vi "Calibration page.vi"(0 "sensor data array":dbl[](array[numeric]), 1 "sensor thr array":dbl[](array[numeric]), 2 "counting role":T1(ring), 3 "sensor1 array":dbl[](array[numeric]), 4 "curv array in":dbl[](array[numeric]), 5 "count in":dbl, 6 "sensor2 array":dbl[](array[numeric]), 7 "sensor3 array":dbl[](array[numeric]), 8 "curv sw info":dbl[](array[numeric]), 9 "capture":bool, 10 "cyrv avg array in":dbl[][][](array[numeric]), 11 "error in":errorcluster, 16 "sen plt num":i32) -> (12 "Left Sidewall":bool, 13 "cyrv avg array out":dbl[][][](array[numeric]), 14 "Right Sidewall":bool, 15 "curv sit":bool, 17 "Boolean Rectangle 5":bool, 18 "Col Curve":dbl[](array[numeric]), 19 "error out":errorcluster, 20 "Curvness Sensors Graph":dynamicdata(graph), 21 "SideWall Sensors Graph":dynamicdata(graph), 22 "sensor1 array out":dbl[](array[numeric]), 23 "curv array out":dbl[](array[numeric]), 24 "sensor2 array out":dbl[](array[numeric]), 25 "sensor3 array out":dbl[](array[numeric]), 26 "capture":bool, 27 "Pallet CURV (mm)":dbl format="%#_2g")   [LabVIEW 2019]
uses:
  <vilib>/measure/mamon.llb/Trigger Detection for 1 Channel.vi
  <vilib>/measure/NI_MAPro.lvlib
panel:
  out "curv array in 2":dbl[](array[numeric])
  out "subarray 3":dbl[](array[numeric])
  out "subarray 2":dbl[](array[numeric])
  out "Boolean":bool
  out "subarray":dbl[](array[numeric])
  out "x+y 3":dbl
  out "x+y 2":dbl
  out "x+y":dbl
  in  "bias":dbl format="%#_13g"
  out "sesor3-2 dis":dbl
  out "sensor2-2 dis":dbl
  out "sensor1-2 dis":dbl
  out "Numeric 3":i32=1
  out "Numeric 2":i32=1
  out "sensor3 dis":dbl
  out "sensor2 dis":dbl
  out "sensor1 dis":dbl
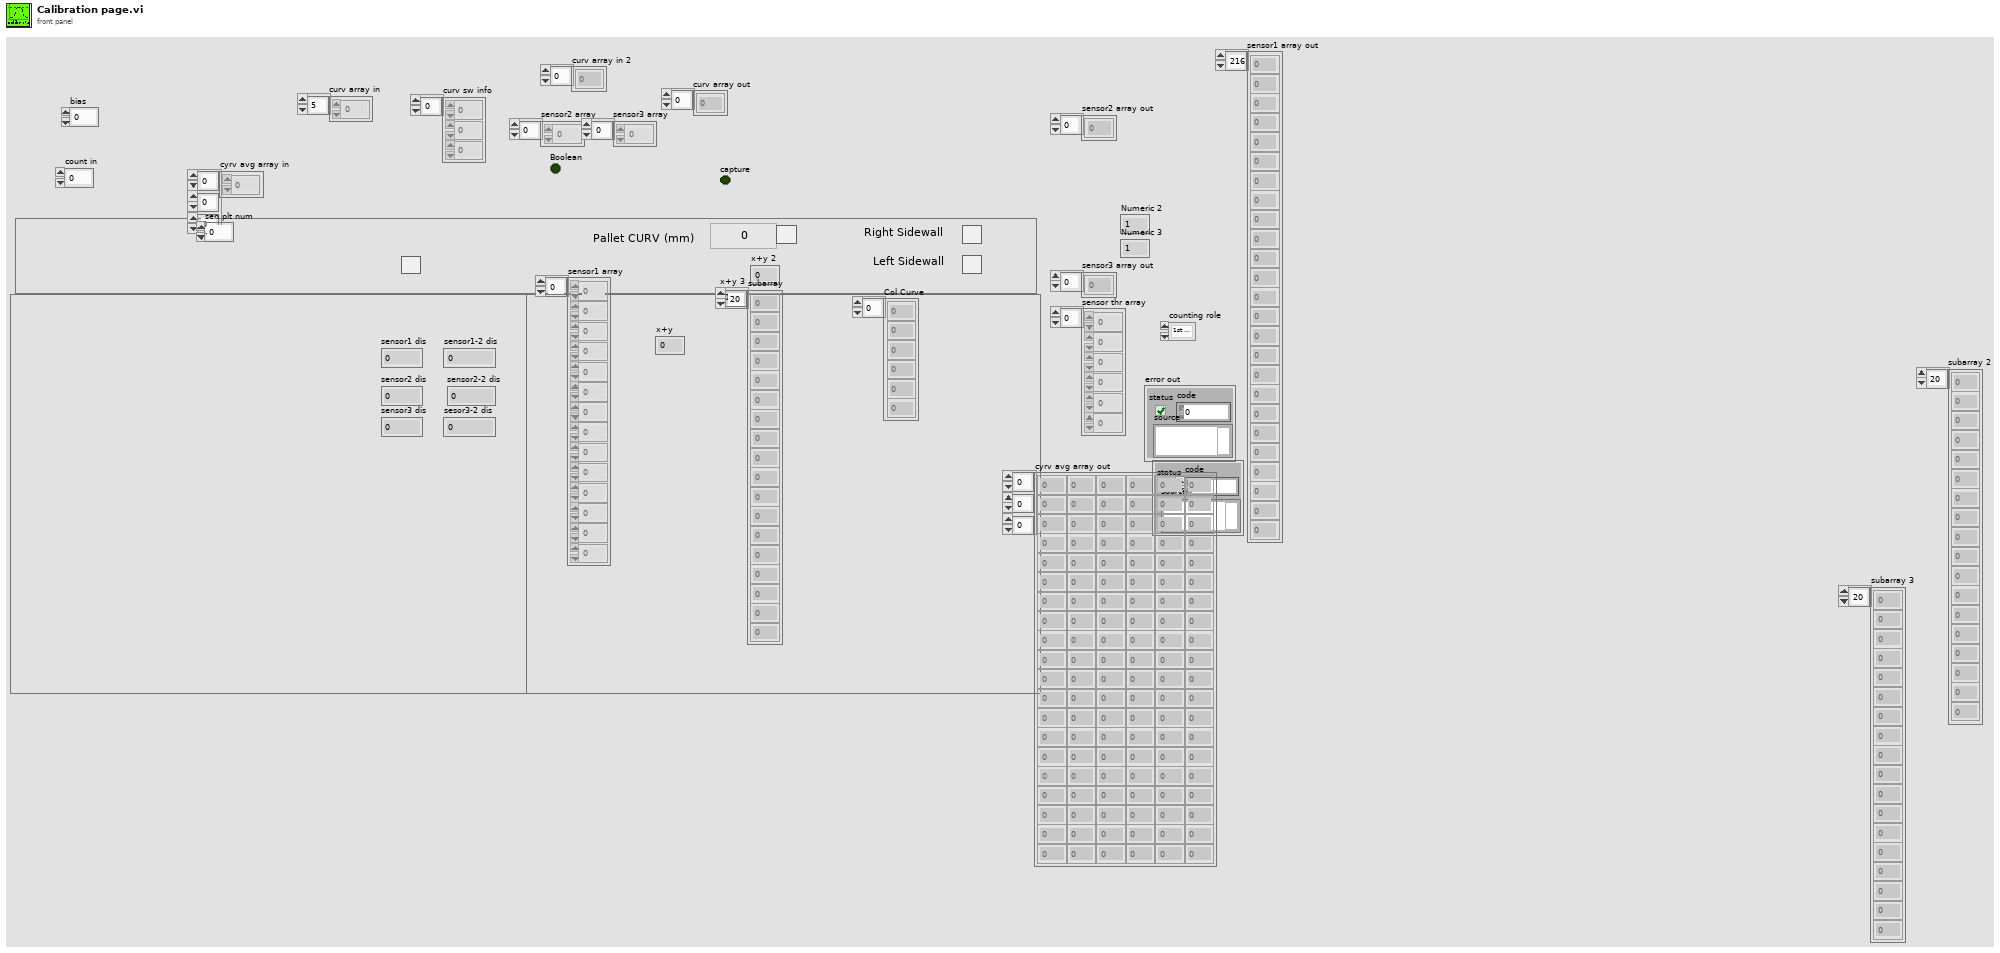
[diagram p1: front panel]
types:
  T1 = enum16{"1st sensor", "2nd sensor", "3rd sensor", "1st+2nd", "1st+3rd", "2nd+3rd", "1st+2nd+3rd"}
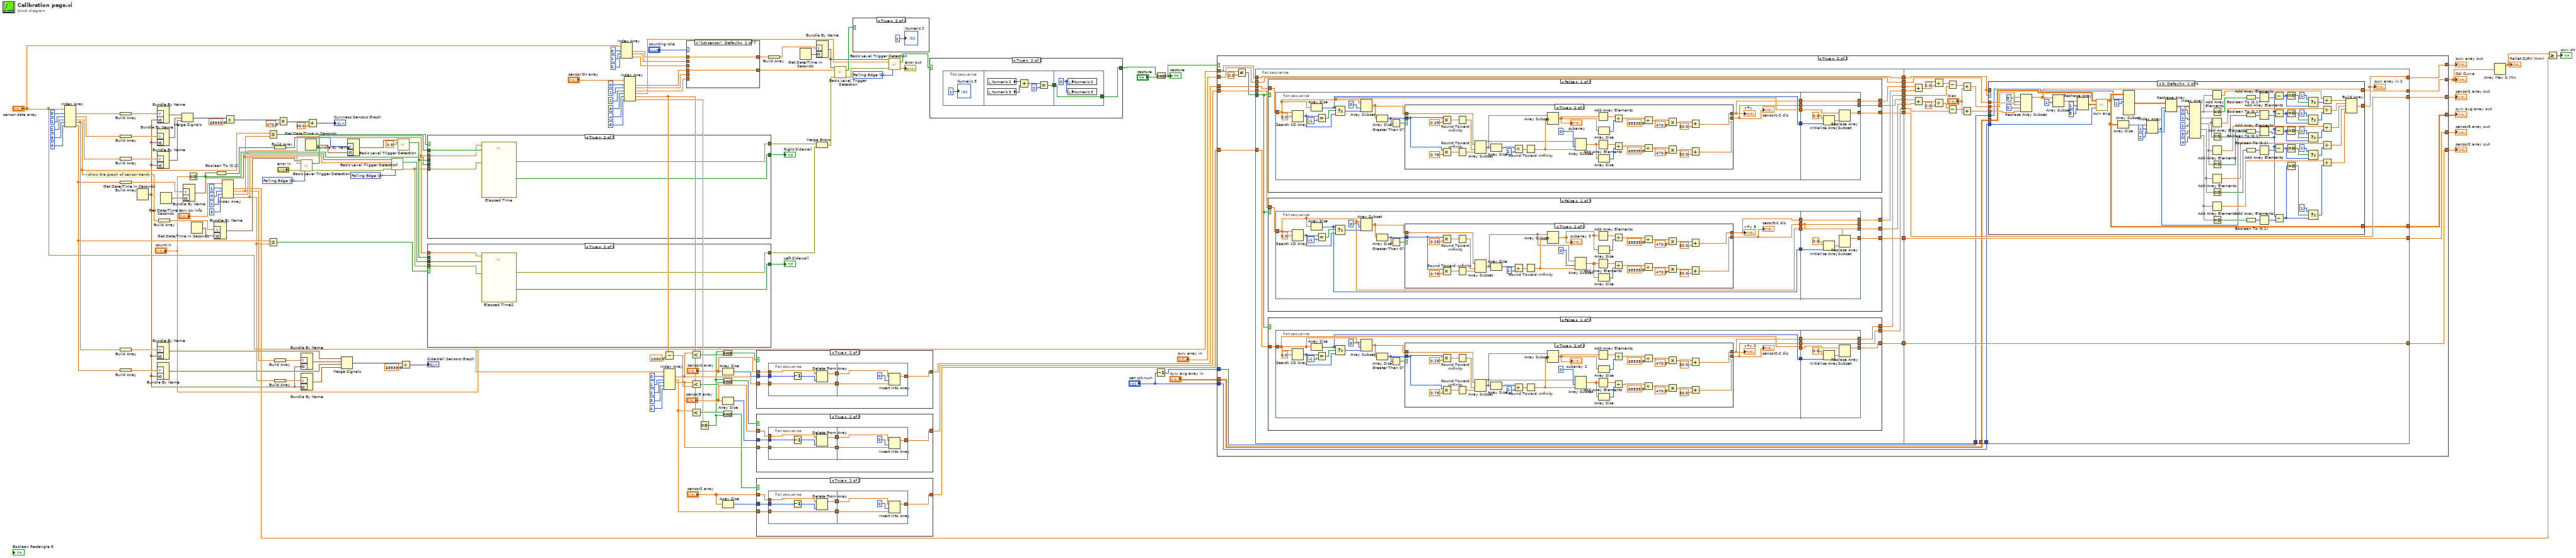
[diagram p0: block diagram]
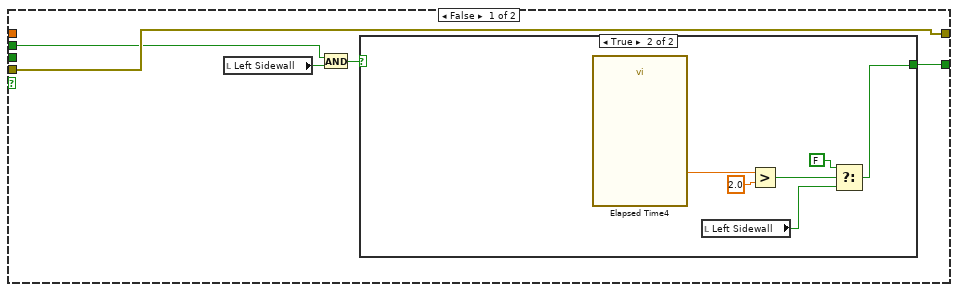
[diagram p5: hidden frame]
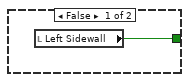
[diagram p6: hidden frame]
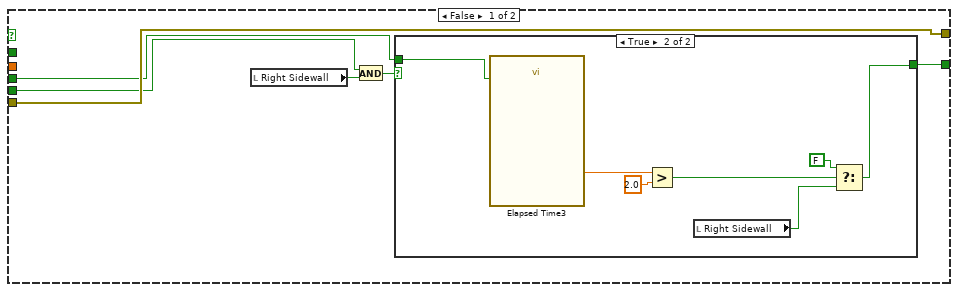
[diagram p7: hidden frame]
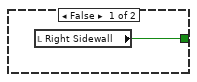
[diagram p8: hidden frame]
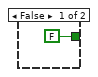
[diagram p9: hidden frame]
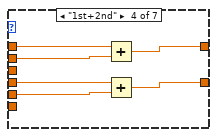
[diagram p13: hidden frame]
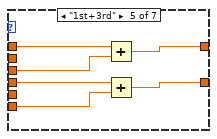
[diagram p14: hidden frame]
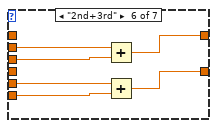
[diagram p15: hidden frame]
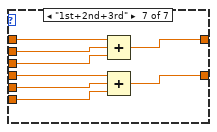
[diagram p16: hidden frame]
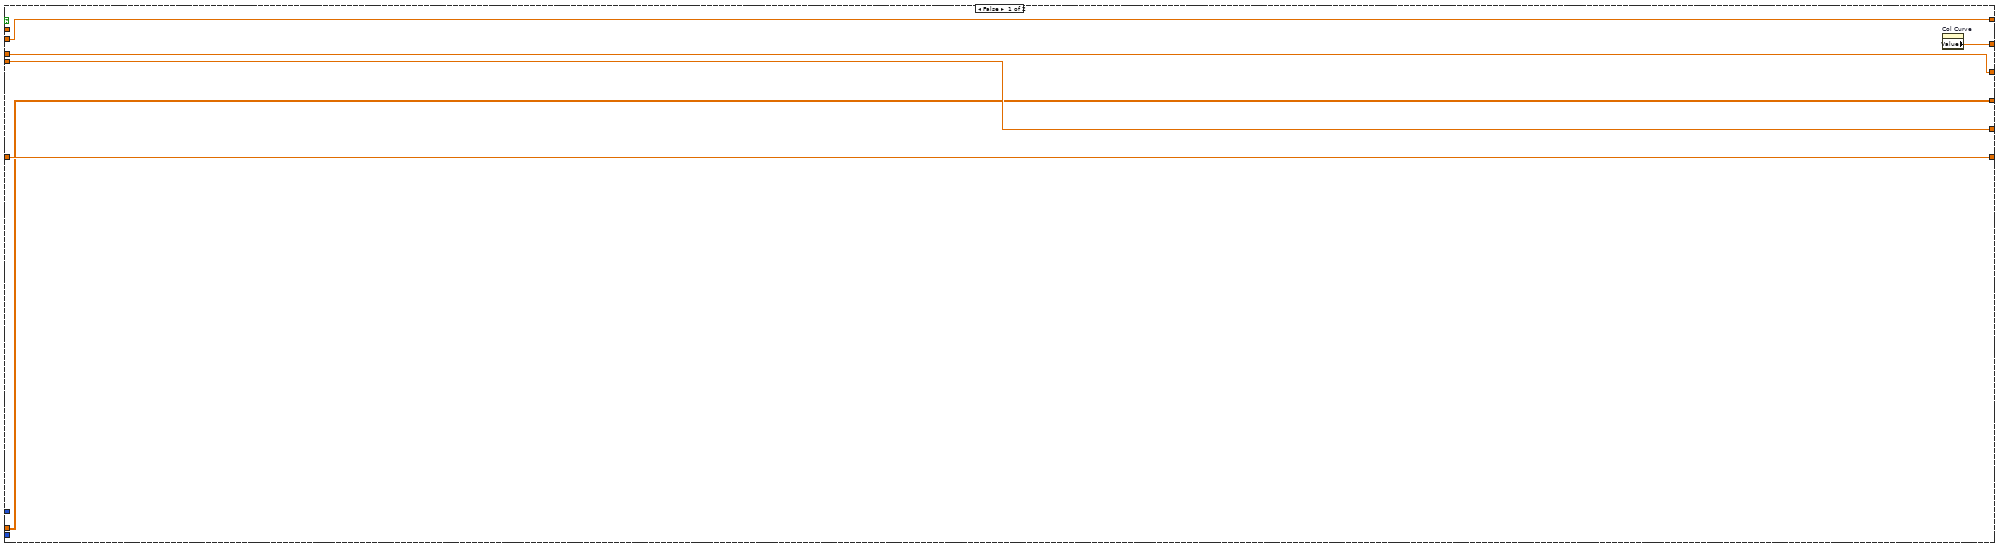
[diagram p17: hidden frame]
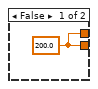
[diagram p18: hidden frame]
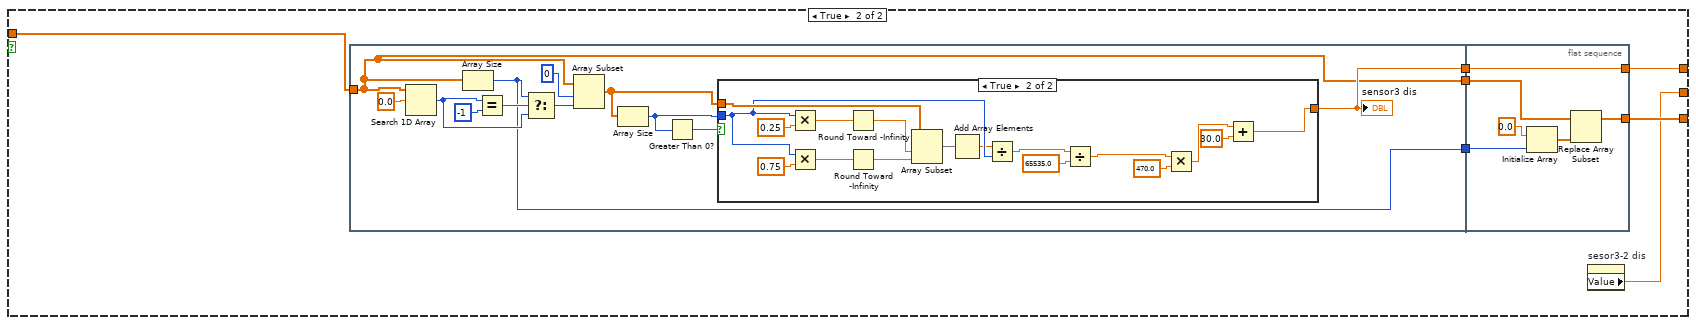
[diagram p19: hidden frame]
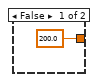
[diagram p20: hidden frame]
diagram:
  w38 = u16 0 items=["Falling Edge", "Rising Edge"] ("trigger slope")
  w39 = u16 0 items=["Falling Edge", "Rising Edge"] ("trigger slope")
  w100 = u16 0 items=["Falling Edge", "Rising Edge"] ("trigger slope")
  # "show the graph of sensor trend"
  n1 = Index Array(array="sensor data array", index #1=0 ("index"), index #2=1 ("index"), index #3=2 ("index"), index #4=3 ("index"), index #5=4 ("index")) -> (element #1=w136:dbl, element #2=w134:dbl, element #3=w132:dbl, element #4=w69:dbl, element #5=w68:dbl)
  n2 = Build Array(w136) -> (w135:dbl[])
  n3 = Build Array(w134) -> (w133:dbl[])
  n4 = Build Array(w132) -> (w131:dbl[])
  n5 = Build Array(w68) -> (w67:dbl[])
  n6 = Build Array(w69) -> (w130:dbl[])
  n7 = Build Array(w68) -> (w129:dbl[])
  n8 = Get Date/Time In Seconds() -> (seconds since 1Jan1904=w12:timestamp)
  n9 = Bundle By Name("Y"=w135, "t0"=w12) -> (w123:waveform(dbl))  [unwired: 1 in]
  n10 = Bundle By Name("Y"=w133, "t0"=w12) -> (w144:waveform(dbl))  [unwired: 1 in]
  n11 = Bundle By Name("Y"=w131, "t0"=w12) -> (w143:waveform(dbl))  [unwired: 1 in]
  n12 = Bundle By Name("Y"=w130, "t0"=w12) -> (w142:waveform(dbl))  [unwired: 1 in]
  n13 = Bundle By Name("Y"=w129, "t0"=w12) -> (w17:waveform(dbl))  [unwired: 1 in]
  n14 = Build Array(w69) -> (w70:dbl[])
  n15 = Get Date/Time In Seconds() -> (seconds since 1Jan1904=w92:timestamp)
  n16 = Merge Signals(w123, w144, w143) -> (w11:dynamicdata)
  n17 = Bundle By Name("Y"=w67, "t0"=w92) -> (w93:waveform(dbl))  [unwired: 1 in]
  n18 = Equal To 0?(x="count in") -> (x = 0?=w28:bool)
  n19 = Get Date/Time In Seconds() -> (seconds since 1Jan1904=w96:timestamp)
  n20 = Bundle By Name("Y"=w70, "t0"=w96) -> (w95:waveform(dbl))  [unwired: 1 in]
  n21 = Boolean To (0,1)(Boolean=w28) -> (0, 1=w32:i16)
  n22 = Index Array(array="curv sw info", index #1=1 ("index"), index #2=0 ("index"), index #3=2 ("index"), index #4=3 ("index")) -> (element #1=w43:dbl, element #2=w19:dbl, element #3=w66:dbl, element #4=w14:dbl)
  n23 = Divide(x=w11, y=65535.0) -> (x/y=w26:dynamicdata)
  n24 = Less Or Equal?(x=w69, y=w19) -> (x <= y?=w98:bool)
  n25 = Less Or Equal?(x=w68, y=w14) -> (x <= y?=w97:bool)
  n26 = Build Array(w32) -> (w31:i16[])
  n27 = Build Array(w19) -> (w18:dbl[])
  n28 = Build Array(w14) -> (w15:dbl[])
  n29 = Multiply(x=w26, y=470.0) -> (x*y=w27:dynamicdata)
  n30 = call-poly <vilib>:"Basic Level Trigger Detection.vi"("signal in"=w95, "level"=w19, "error in (no error)"="error in", "trigger slope"=w39) -> ("trigger detected?"=w94:bool, "error out"=w89:errorcluster)  [unwired: 9 in, 1 out]
  n31 = Bundle By Name("Y"=w18, "t0"=w12) -> (w16:waveform(dbl))  [unwired: 1 in]
  n32 = Bundle By Name("Y"=w15, "t0"=w12) -> (w13:waveform(dbl))  [unwired: 1 in]
  n33 = Get Date/Time In Seconds() -> (seconds since 1Jan1904=w33:timestamp)
  n34 = Add(x=w27, y=30.0) -> (x+y=→"Curvness Sensors Graph":dynamicdata)
  n35 = Merge Signals(w142, w16, w17, w13) -> (w21:dynamicdata)
  n36 = Bundle By Name("Y"=w31, "t0"=w33) -> (w34:waveform(i16))  [unwired: 1 in]
  n37 = call-poly <vilib>:"Basic Level Trigger Detection.vi"("signal in"=w93, "level"=w14, "error in (no error)"=w89, "trigger slope"=w38) -> ("trigger detected?"=w91:bool, "error out"=w51:errorcluster)  [unwired: 9 in, 1 out]
  n38 = call-poly <vilib>:"Basic Level Trigger Detection.vi"("signal in"=w34, "level"=0.5) -> ("trigger detected?"=w29:bool)  [unwired: 11 in, 2 out]
  n39 = Divide(x=w21, y=65535.0) -> (x/y=→"SideWall Sensors Graph":dynamicdata)
  n40 = case shown="True" w98 {
    tunnel: w94 -> [_ w163]
    tunnel: w66 -> [_ w162]
    tunnel: w51 -> [w150 w161]
    tunnel: [w150 w160] -> w50
    tunnel: [w149 w159] -> w37
    tunnel: w29 -> [w148 _]
    tunnel: w28 -> [w146 _]
    frame False {
      n41 = local read "Right Sidewall"() -> (w147:bool)
      n42 = And(x=w146, y=w147) -> (x .and. y?=w145:bool)
      n43 = case shown="True" w145 {
        tunnel: [w151 w153] -> w149
        tunnel: w148 -> [_ w152]
        frame False {
          n44 = local read "Right Sidewall"() -> (w151:bool)
        }
        frame True {
          n45 = call "Elapsed Time3"("Reset"=w152) -> ("Elapsed Time (s)"=w158:dbl)  [unwired: 11 in, 7 out]
          n46 = Greater?(x=w158, y=2.0) -> (0:w156:bool)
          n47 = local read "Right Sidewall"() -> (w154:bool)
          n48 = Select(t=FALSE, s=w156, f=w154) -> (s? t:f=w153:bool)
        }
      }
    }
    frame True {
      n49 = call "Elapsed Time"("Time Target (s)"=w162, "Reset"=w163, "error in (no error)"=w161) -> ("Time has Elapsed"=w159:bool, "error out"=w160:errorcluster)  [unwired: 9 in, 6 out]
    }
  }
  "Right Sidewall" <- w37
  n50 = case shown="True" w97 {
    tunnel: w91 -> [_ w180]
    tunnel: w66 -> [_ w179]
    tunnel: w51 -> [w168 w178]
    tunnel: [w168 w177] -> w49
    tunnel: [w167 w176] -> w36
    tunnel: w29 -> [w165 _]
    frame False {
      n51 = local read "Left Sidewall"() -> (w166:bool)
      n52 = And(x=w165, y=w166) -> (x .and. y?=w164:bool)
      n53 = case shown="True" w164 {
        tunnel: [w169 w170] -> w167
        frame False {
          n54 = local read "Left Sidewall"() -> (w169:bool)
        }
        frame True {
          n55 = call "Elapsed Time4"() -> ("Elapsed Time (s)"=w171:dbl)  [unwired: 12 in, 7 out]
          n56 = local read "Left Sidewall"() -> (w172:bool)
          n57 = Greater?(x=w171, y=2.0) -> (0:w174:bool)
          n58 = Select(t=FALSE, s=w174, f=w172) -> (s? t:f=w170:bool)
        }
      }
    }
    frame True {
      n59 = call "Elapsed Time2"("Time Target (s)"=w179, "Reset"=w180, "error in (no error)"=w178) -> ("Time has Elapsed"=w176:bool, "error out"=w177:errorcluster)  [unwired: 9 in, 6 out]
    }
  }
  "Left Sidewall" <- w36
  n60 = Index Array(array="sensor data array", index #1=0 ("index"), index #2=1 ("index"), index #3=2 ("index")) -> (element #1=w111:dbl, element #2=w110:dbl, element #3=w109:dbl)
  n61 = Index Array(array="sensor thr array", index #1=0 ("index"), index #2=1 ("index"), index #3=2 ("index"), index #4=3 ("index"), index #5=4 ("index"), index #6=6 ("index")) -> (element #1=w117:dbl, element #2=w116:dbl, element #3=w115:dbl, element #4=w56:dbl, element #5=w55:dbl, element #6=w9:dbl)
  n62 = Subtract(x=w55, y=1000.0) -> (x-y=w53:dbl)
  n63 = Index Array(array="sensor data array", index #1=0 ("index"), index #2=1 ("index"), index #3=2 ("index"), index #4=3 ("index"), index #5=4 ("index")) -> (element #1=w77:dbl, element #2=w76:dbl, element #3=w75:dbl)  [unwired: 2 out]
  n64 = case shown="\"1st sensor\", Default" "counting role" {
    tunnel: w111 -> [w182 _ _ w190 w198 _ w212]
    tunnel: w117 -> [w181 _ _ w191 w196 _ w209]
    tunnel: w110 -> [_ w184 _ w192 _ w204 w211]
    tunnel: w109 -> [_ _ w186 _ w197 w203 w210]
    tunnel: w116 -> [_ w183 _ w189 _ w202 w208]
    tunnel: w115 -> [_ _ w185 _ w195 w201 w207]
    tunnel: [w182 w184 w186 w188 w194 w200 w206] -> w105
    tunnel: [w181 w183 w185 w187 w193 w199 w205] -> w106
    frame "1st sensor", Default {
    }
    frame "2nd sensor" {
    }
    frame "3rd sensor" {
    }
    frame "1st+2nd" {
      n65 = Add(x=w190, y=w192) -> (x+y=w188:dbl)
      n66 = Add(x=w191, y=w189) -> (x+y=w187:dbl)
    }
    frame "1st+3rd" {
      n67 = Add(x=w198, y=w197) -> (x+y=w194:dbl)
      n68 = Add(x=w196, y=w195) -> (x+y=w193:dbl)
    }
    frame "2nd+3rd" {
      n69 = Add(x=w204, y=w203) -> (x+y=w200:dbl)
      n70 = Add(x=w202, y=w201) -> (x+y=w199:dbl)
    }
    frame "1st+2nd+3rd" {
      n71 = Compound Arithmetic op=ADD(w212, w211, w210) -> (w206:dbl)
      n72 = Compound Arithmetic op=ADD(w209, w208, w207) -> (w205:dbl)
    }
  }
  n73 = Less?(x=w77, y=w55) -> (x < y?=w8:bool)
  n74 = Less?(x=w75, y=w53) -> (x < y?=w4:bool)
  n75 = Less?(x=w76, y=w55) -> (x < y?=w6:bool)
  n76 = Equal To 0?(x=w9) -> (x = 0?=w3:bool)
  n77 = And(x=w3, y=w8) -> (x .and. y?=w7:bool)
  n78 = And(x=w3, y=w4) -> (x .and. y?=w2:bool)
  n79 = And(x=w6, y=w3) -> (x .and. y?=w5:bool)
  n80 = Array Size(array="sensor1 array") -> (size(s)=w81:i32)
  n81 = Array Size(array="sensor3 array") -> (size(s)=w78:i32)
  n82 = Array Size(array="sensor2 array") -> (size(s)=w80:i32)
  n83 = case shown="True" w7 {
    tunnel: w77 -> [_ w214]
    tunnel: "sensor1 array" -> [w213 w219]
    tunnel: w81 -> [_ w218]
    tunnel: [w213 w216] -> w62
    frame False {
    }
    frame True {
      n84 = flat-sequence {
        tunnel: w219 -> [w224]
        tunnel: w218 -> [w223]
        tunnel: [w221] -> w217
        tunnel: [w220] -> w215
        tunnel: w214 -> [w220]
        tunnel: [w228] -> w216
        tunnel: w215 -> [w225]
        tunnel: w217 -> [w227]
        frame #0 {
          n85 = Decrement(x=w223) -> (x-1=w222:i32)
          n86 = Delete From Array(array=w224, index=w222) -> (array with subset deleted=w221:dbl[])  [unwired: 1 in, 1 out]
        }
        frame #1 {
          n87 = Insert Into Array(array=w227, index=0, new element=w225) -> (w228:dbl[])
        }
      }
    }
  }
  n88 = case shown="True" w2 {
    tunnel: w75 -> [_ w235]
    tunnel: "sensor3 array" -> [w229 w234]
    tunnel: w78 -> [_ w233]
    tunnel: [w229 w230] -> w60
    frame False {
    }
    frame True {
      n89 = flat-sequence {
        tunnel: w235 -> [w236]
        tunnel: w234 -> [w239]
        tunnel: w233 -> [w238]
        tunnel: [w237] -> w232
        tunnel: [w236] -> w231
        tunnel: w232 -> [w243]
        tunnel: w231 -> [w242]
        tunnel: [w241] -> w230
        frame #0 {
          n90 = Decrement(x=w238) -> (x-1=w240:i32)
          n91 = Delete From Array(array=w239, index=w240) -> (array with subset deleted=w237:dbl[])  [unwired: 1 in, 1 out]
        }
        frame #1 {
          n92 = Insert Into Array(array=w243, index=0, new element=w242) -> (w241:dbl[])
        }
      }
    }
  }
  n93 = case shown="True" w5 {
    tunnel: w76 -> [_ w251]
    tunnel: "sensor2 array" -> [w245 w250]
    tunnel: w80 -> [_ w249]
    tunnel: [w245 w246] -> w61
    frame False {
    }
    frame True {
      n94 = flat-sequence {
        tunnel: w251 -> [w252]
        tunnel: w250 -> [w255]
        tunnel: w249 -> [w254]
        tunnel: [w253] -> w248
        tunnel: [w252] -> w247
        tunnel: w248 -> [w259]
        tunnel: w247 -> [w258]
        tunnel: [w257] -> w246
        frame #0 {
          n95 = Decrement(x=w254) -> (x-1=w256:i32)
          n96 = Delete From Array(array=w255, index=w256) -> (array with subset deleted=w253:dbl[])  [unwired: 1 in, 1 out]
        }
        frame #1 {
          n97 = Insert Into Array(array=w259, index=0, new element=w258) -> (w257:dbl[])
        }
      }
    }
  }
  n98 = Build Array(w105) -> (w108:dbl[])
  n99 = Get Date/Time In Seconds() -> (seconds since 1Jan1904=w107:timestamp)
  n100 = Bundle By Name("Y"=w108, "t0"=w107) -> (w104:waveform(dbl))  [unwired: 1 in]
  n101 = Merge Errors(w50, w49) -> (w48:errorcluster)
  n102 = call-poly <vilib>:"Basic Level Trigger Detection.vi"("signal in"=w104, "level"=w106, "error in (no error)"=w48) -> ("trigger detected?"=w103:bool, "error out"=w101:errorcluster)  [unwired: 10 in, 1 out]
  n103 = case shown="True" w103 {
    frame False {
    }
    frame True {
      "Numeric 2" <- 1
    }
  }
  n104 = call-poly <vilib>:"Basic Level Trigger Detection.vi"("signal in"=w104, "level"=w56, "error in (no error)"=w101, "trigger slope"=w100) -> ("trigger detected?"=w102:bool, "error out"=→"error out":errorcluster)  [unwired: 9 in, 1 out]
  n105 = case shown="True" w102 {
    tunnel: [FALSE w264] -> w88
    frame False {
    }
    frame True {
      n106 = flat-sequence {
        tunnel: [w266] -> w263
        tunnel: [w272] -> w264
        tunnel: w263 -> [w272]
        frame #0 {
          "Numeric 3" <- 1
        }
        frame #1 {
          n107 = local read "Numeric 2"() -> (w270:i32)
          n108 = local read "Numeric 3"() -> (w269:i32)
          n109 = Add(x=w270, y=w269) -> (x+y=w268:i32)
          n110 = Equal?(x=w268, y=2) -> (x = y?=w266:bool)
        }
        frame #2 {
          w271 = 0 ("Numeric")
          n111 = local write "Numeric 2"(w271) -> ()
          n112 = local write "Numeric 3"(w271) -> ()
        }
      }
    }
  }
  n113 = Decrement(x="sen plt num") -> (x-1=w42:i32)
  n114 = And(x=w88, y="capture") -> (x .and. y?=w84:bool)
  "capture" <- w84
  n115 = case shown="True" w84 {
    tunnel: "count in" -> [_ w302]
    tunnel: "curv array in" -> [w278 w305]
    tunnel: [w278 w298] -> w83
    tunnel: w62 -> [w277 w301]
    tunnel: w61 -> [w276 w297]
    tunnel: w60 -> [w275 w296]
    tunnel: [w277 w288] -> w65
    tunnel: [w276 w286] -> w64
    tunnel: [w275 w284] -> w63
    tunnel: "cyrv avg array in" -> [w274 w283]
    tunnel: [w274 w282] -> w45
    tunnel: "sen plt num" -> [_ w281]
    tunnel: w42 -> [_ w279]
    tunnel: [w273 w280] -> w41
    frame False {
      n116 = property on="Col Curve" class="Arr (strict)"() -> ("Value"=w273:dbl[])  [unwired: 2 in, 2 out]
    }
    frame True {
      n117 = Not Equal?(x=w302, y=0.0) -> (x != y?=w303:bool)
      n118 = flat-sequence {
        tunnel: w302 -> [w320]
        tunnel: w305 -> [w319]
        tunnel: w303 -> [w316]
        tunnel: w301 -> [w318]
        tunnel: [w320] -> w300
        tunnel: [w319] -> w299
        tunnel: w297 -> [w317]
        tunnel: w296 -> [w315]
        tunnel: [w314] -> w295
        tunnel: [w313] -> w294
        tunnel: [w312] -> w293
        tunnel: [w311] -> w292
        tunnel: [w310] -> w291
        tunnel: [w309] -> w290
        tunnel: [w308] -> w289
        tunnel: [w307] -> w287
        tunnel: [w306] -> w285
        tunnel: w300 -> [w661]
        tunnel: w299 -> [w660]
        tunnel: [w662] -> w298
        tunnel: w295 -> [w659]
        tunnel: w294 -> [w642]
        tunnel: w293 -> [w640]
        tunnel: w292 -> [w658]
        tunnel: w291 -> [w641]
        tunnel: w290 -> [w639]
        tunnel: w289 -> [w657]
        tunnel: [w657] -> w288
        tunnel: w287 -> [w656]
        tunnel: [w656] -> w286
        tunnel: w285 -> [w655]
        tunnel: [w655] -> w284
        tunnel: w283 -> [w647]
        tunnel: [w646] -> w282
        tunnel: w281 -> [w645]
        tunnel: [w644] -> w280
        tunnel: w279 -> [w643]
        frame #0 {
          n119 = case shown="False" w316 {
            tunnel: w318 -> [w540 w602]
            tunnel: [w538 w599] -> w308
            tunnel: [w536 w598] -> w314
            tunnel: [w534 w596] -> w311
            frame False {
              n120 = flat-sequence {
                tunnel: w540 -> [w548]
                tunnel: [w548] -> w539
                tunnel: [w547] -> w537
                tunnel: [w542] -> w535
                tunnel: [w543] -> w533
                tunnel: w539 -> [w593]
                tunnel: [w592] -> w538
                tunnel: w537 -> [w591]
                tunnel: [w590] -> w536
                tunnel: w535 -> [w590]
                tunnel: [w589] -> w534
                tunnel: w533 -> [w589]
                frame #0 {
                  n121 = Search 1D Array(1D array=w548, element=0.0) -> (index of element=w546:i32)  [unwired: 1 in]
                  n122 = Array Size(array=w548) -> (size(s)=w547:i32)
                  n123 = Equal?(x=w546, y=-1) -> (x = y?=w550:bool)
                  n124 = Select(t=w547, s=w550, f=w546) -> (s? t:f=w549:i32)
                  n125 = Array Subset(array=w548, index=0, length=w549) -> (w545:dbl[])
                  n126 = Array Size(array=w545) -> (size(s)=w544:i32)
                  n127 = Greater Than 0?(x=w544) -> (x > 0?=w541:bool)
                  n128 = case shown="True" w541 {
                    tunnel: w545 -> [_ w560]
                    tunnel: w544 -> [_ w557]
                    tunnel: [w554 w556] -> w543
                    tunnel: [w554 w555] -> w542
                    frame False {
                      w554 = 200.0
                    }
                    frame True {
                      n129 = Multiply(x=w557, y=0.25) -> (x*y=w566:dbl)
                      n130 = Multiply(x=w557, y=0.75) -> (x*y=w564:dbl)
                      n131 = Round Toward -Infinity(1:w566) -> (0:w565:dbl)
                      n132 = Round Toward -Infinity(1:w564) -> (0:w563:dbl)
                      n133 = Array Subset(array=w560, index=w565, length=w563) -> (w559:dbl[])
                      n134 = Array Size(array=w559) -> (size(s)=w558:i32)
                      n135 = Divide(x=w558, y=2) -> (x/y=w568:dbl)
                      n136 = Round Toward -Infinity(1:w568) -> (0:w567:dbl)
                      n137 = Array Subset(array=w559, index=w567) -> (w580:dbl[])  [unwired: 1 in]
                      "subarray" <- w580
                      n138 = Array Subset(array=w559, index=0, length=w567) -> (w572:dbl[])
                      n139 = Add Array Elements(numeric array=w580) -> (sum=w585:dbl)
                      n140 = Add Array Elements(numeric array=w572) -> (sum=w576:dbl)
                      n141 = Array Size(array=w580) -> (size(s)=w570:i32)
                      n142 = Array Size(array=w572) -> (size(s)=w569:i32)
                      n143 = Divide(x=w585, y=w570) -> (x/y=w586:dbl)
                      n144 = Divide(x=w576, y=w569) -> (x/y=w575:dbl)
                      n145 = Divide(x=w586, y=65535.0) -> (x/y=w587:dbl)
                      n146 = Divide(x=w575, y=65535.0) -> (x/y=w574:dbl)
                      n147 = Multiply(x=w587, y=470.0) -> (x*y=w588:dbl)
                      n148 = Multiply(x=w574, y=470.0) -> (x*y=w573:dbl)
                      n149 = Add(x=w588, y=30.0) -> (x+y=w555:dbl)
                      n150 = Add(x=w573, y=30.0) -> (x+y=w556:dbl)
                    }
                  }
                  "sensor1-2 dis" <- w543
                  "x+y" <- w542
                }
                frame #1 {
                  n151 = Initialize Array(0.0 ("element"), w591) -> (w594:dbl[])
                  n152 = Replace Array Subset(array=w593, new element=w594) -> (w592:dbl[])  [unwired: 1 in]
                }
              }
            }
            frame True {
              n153 = flat-sequence {
                tunnel: w602 -> [w608]
                tunnel: [w609] -> w601
                tunnel: [w608] -> w600
                tunnel: [w604] -> w597
                tunnel: w601 -> [w637]
                tunnel: w600 -> [w636]
                tunnel: [w634] -> w599
                tunnel: [w633] -> w598
                tunnel: w597 -> [w633]
                frame #0 {
                  n154 = Search 1D Array(1D array=w608, element=0.0) -> (index of element=w607:i32)  [unwired: 1 in]
                  n155 = Array Size(array=w608) -> (size(s)=w609:i32)
                  n156 = Equal?(x=w607, y=-1) -> (x = y?=w611:bool)
                  n157 = Select(t=w609, s=w611, f=w607) -> (s? t:f=w610:i32)
                  n158 = Array Subset(array=w608, index=0, length=w610) -> (w606:dbl[])
                  n159 = Array Size(array=w606) -> (size(s)=w605:i32)
                  n160 = Greater Than 0?(x=w605) -> (x > 0?=w603:bool)
                  n161 = case shown="True" w603 {
                    tunnel: w606 -> [_ w632]
                    tunnel: w605 -> [_ w631]
                    tunnel: [200.0 w616] -> w604
                    frame False {
                    }
                    frame True {
                      n162 = Multiply(x=w631, y=0.25) -> (x*y=w622:dbl)
                      n163 = Multiply(x=w631, y=0.75) -> (x*y=w620:dbl)
                      n164 = Round Toward -Infinity(1:w622) -> (0:w621:dbl)
                      n165 = Round Toward -Infinity(1:w620) -> (0:w618:dbl)
                      n166 = Array Subset(array=w632, index=w621, length=w618) -> (w617:dbl[])
                      n167 = Add Array Elements(numeric array=w617) -> (sum=w627:dbl)
                      n168 = Divide(x=w627, y=w631) -> (x/y=w628:dbl)
                      n169 = Divide(x=w628, y=65535.0) -> (x/y=w629:dbl)
                      n170 = Multiply(x=w629, y=470.0) -> (x*y=w630:dbl)
                      n171 = Add(x=w630, y=30.0) -> (x+y=w616:dbl)
                    }
                  }
                  "sensor1 dis" <- w604
                }
                frame #1 {
                  n172 = Initialize Array(0.0 ("element"), w637) -> (w635:dbl[])
                  n173 = Replace Array Subset(array=w636, new element=w635) -> (w634:dbl[])  [unwired: 1 in]
                }
              }
              n174 = property on="sensor1-2 dis" class="DigNum (strict)"() -> ("Value"=w596:dbl)  [unwired: 2 in, 2 out]
            }
          }
          n175 = case shown="False" w316 {
            tunnel: w315 -> [w328 w390]
            tunnel: [w327 w387] -> w306
            tunnel: [w321 w386] -> w313
            tunnel: [w322 w384] -> w310
            frame False {
              n176 = flat-sequence {
                tunnel: w328 -> [w332]
                tunnel: [w330] -> w326
                tunnel: [w329] -> w325
                tunnel: [w331] -> w324
                tunnel: [w332] -> w323
                tunnel: [w381] -> w327
                tunnel: [w377] -> _
                tunnel: w326 -> [w377]
                tunnel: [w378] -> w321
                tunnel: w325 -> [w378]
                tunnel: w324 -> [w379]
                tunnel: w323 -> [w380]
                tunnel: [w377] -> w322
                frame #0 {
                  n177 = Search 1D Array(1D array=w332, element=0.0) -> (index of element=w336:i32)  [unwired: 1 in]
                  n178 = Array Size(array=w332) -> (size(s)=w331:i32)
                  n179 = Equal?(x=w336, y=-1) -> (x = y?=w338:bool)
                  n180 = Select(t=w331, s=w338, f=w336) -> (s? t:f=w337:i32)
                  n181 = Array Subset(array=w332, index=0, length=w337) -> (w335:dbl[])
                  n182 = Array Size(array=w335) -> (size(s)=w334:i32)
                  n183 = Greater Than 0?(x=w334) -> (x > 0?=w333:bool)
                  n184 = case shown="True" w333 {
                    tunnel: w335 -> [_ w348]
                    tunnel: w334 -> [_ w345]
                    tunnel: [w342 w344] -> w330
                    tunnel: [w342 w343] -> w329
                    frame False {
                      w342 = 200.0
                    }
                    frame True {
                      n185 = Multiply(x=w345, y=0.25) -> (x*y=w354:dbl)
                      n186 = Multiply(x=w345, y=0.75) -> (x*y=w352:dbl)
                      n187 = Round Toward -Infinity(1:w354) -> (0:w353:dbl)
                      n188 = Round Toward -Infinity(1:w352) -> (0:w351:dbl)
                      n189 = Array Subset(array=w348, index=w353, length=w351) -> (w347:dbl[])
                      n190 = Array Size(array=w347) -> (size(s)=w346:i32)
                      n191 = Divide(x=w346, y=2) -> (x/y=w356:dbl)
                      n192 = Round Toward -Infinity(1:w356) -> (0:w355:dbl)
                      n193 = Array Subset(array=w347, index=w355) -> (w368:dbl[])  [unwired: 1 in]
                      "subarray 3" <- w368
                      n194 = Array Subset(array=w347, index=0, length=w355) -> (w360:dbl[])
                      n195 = Add Array Elements(numeric array=w368) -> (sum=w373:dbl)
                      n196 = Add Array Elements(numeric array=w360) -> (sum=w364:dbl)
                      n197 = Array Size(array=w368) -> (size(s)=w358:i32)
                      n198 = Array Size(array=w360) -> (size(s)=w357:i32)
                      n199 = Divide(x=w373, y=w358) -> (x/y=w374:dbl)
                      n200 = Divide(x=w364, y=w357) -> (x/y=w363:dbl)
                      n201 = Divide(x=w374, y=65535.0) -> (x/y=w375:dbl)
                      n202 = Divide(x=w363, y=65535.0) -> (x/y=w362:dbl)
                      n203 = Multiply(x=w375, y=470.0) -> (x*y=w376:dbl)
                      n204 = Multiply(x=w362, y=470.0) -> (x*y=w361:dbl)
                      n205 = Add(x=w376, y=30.0) -> (x+y=w343:dbl)
                      n206 = Add(x=w361, y=30.0) -> (x+y=w344:dbl)
                    }
                  }
                  "sesor3-2 dis" <- w330
                  "x+y 3" <- w329
                }
                frame #1 {
                  n207 = Initialize Array(0.0 ("element"), w379) -> (w382:dbl[])
                  n208 = Replace Array Subset(array=w380, new element=w382) -> (w381:dbl[])  [unwired: 1 in]
                }
              }
            }
            frame True {
              n209 = flat-sequence {
                tunnel: w390 -> [w391]
                tunnel: [w391] -> w389
                tunnel: [w393] -> w388
                tunnel: [w392] -> w385
                tunnel: w389 -> [w424]
                tunnel: w388 -> [w423]
                tunnel: [w422] -> w387
                tunnel: [w421] -> w386
                tunnel: w385 -> [w421]
                frame #0 {
                  n210 = Search 1D Array(1D array=w391, element=0.0) -> (index of element=w397:i32)  [unwired: 1 in]
                  n211 = Array Size(array=w391) -> (size(s)=w393:i32)
                  n212 = Equal?(x=w397, y=-1) -> (x = y?=w399:bool)
                  n213 = Select(t=w393, s=w399, f=w397) -> (s? t:f=w398:i32)
                  n214 = Array Subset(array=w391, index=0, length=w398) -> (w396:dbl[])
                  n215 = Array Size(array=w396) -> (size(s)=w395:i32)
                  n216 = Greater Than 0?(x=w395) -> (x > 0?=w394:bool)
                  n217 = case shown="True" w394 {
                    tunnel: w396 -> [_ w420]
                    tunnel: w395 -> [_ w419]
                    tunnel: [200.0 w404] -> w392
                    frame False {
                    }
                    frame True {
                      n218 = Multiply(x=w419, y=0.25) -> (x*y=w410:dbl)
                      n219 = Multiply(x=w419, y=0.75) -> (x*y=w408:dbl)
                      n220 = Round Toward -Infinity(1:w410) -> (0:w409:dbl)
                      n221 = Round Toward -Infinity(1:w408) -> (0:w406:dbl)
                      n222 = Array Subset(array=w420, index=w409, length=w406) -> (w405:dbl[])
                      n223 = Add Array Elements(numeric array=w405) -> (sum=w415:dbl)
                      n224 = Divide(x=w415, y=w419) -> (x/y=w416:dbl)
                      n225 = Divide(x=w416, y=65535.0) -> (x/y=w417:dbl)
                      n226 = Multiply(x=w417, y=470.0) -> (x*y=w418:dbl)
                      n227 = Add(x=w418, y=30.0) -> (x+y=w404:dbl)
                    }
                  }
                  "sensor3 dis" <- w392
                }
                frame #1 {
                  n228 = Initialize Array(0.0 ("element"), w423) -> (w425:dbl[])
                  n229 = Replace Array Subset(array=w424, new element=w425) -> (w422:dbl[])  [unwired: 1 in]
                }
              }
              n230 = property on="sesor3-2 dis" class="DigNum (strict)"() -> ("Value"=w384:dbl)  [unwired: 2 in, 2 out]
            }
          }
          n231 = case shown="False" w316 {
            tunnel: w317 -> [w434 w496]
            tunnel: [w433 w493] -> w307
            tunnel: [w427 w491] -> w312
            tunnel: [w428 w490] -> w309
            frame False {
              n232 = flat-sequence {
                tunnel: w434 -> [w438]
                tunnel: [w436] -> w432
                tunnel: [w435] -> w431
                tunnel: [w437] -> w430
                tunnel: [w438] -> w429
                tunnel: [w485] -> w433
                tunnel: [w484] -> w428
                tunnel: w432 -> [w484]
                tunnel: w431 -> [w483]
                tunnel: [w483] -> w427
                tunnel: w430 -> [w487]
                tunnel: w429 -> [w486]
                frame #0 {
                  n233 = Search 1D Array(1D array=w438, element=0.0) -> (index of element=w442:i32)  [unwired: 1 in]
                  n234 = Array Size(array=w438) -> (size(s)=w437:i32)
                  n235 = Equal?(x=w442, y=-1) -> (x = y?=w444:bool)
                  n236 = Select(t=w437, s=w444, f=w442) -> (s? t:f=w443:i32)
                  n237 = Array Subset(array=w438, index=0, length=w443) -> (w441:dbl[])
                  n238 = Array Size(array=w441) -> (size(s)=w440:i32)
                  n239 = Greater Than 0?(x=w440) -> (x > 0?=w439:bool)
                  n240 = case shown="True" w439 {
                    tunnel: w441 -> [_ w454]
                    tunnel: w440 -> [_ w451]
                    tunnel: [w448 w450] -> w436
                    tunnel: [w448 w449] -> w435
                    frame False {
                      w448 = 200.0
                    }
                    frame True {
                      n241 = Multiply(x=w451, y=0.25) -> (x*y=w460:dbl)
                      n242 = Multiply(x=w451, y=0.75) -> (x*y=w458:dbl)
                      n243 = Round Toward -Infinity(1:w460) -> (0:w459:dbl)
                      n244 = Round Toward -Infinity(1:w458) -> (0:w457:dbl)
                      n245 = Array Subset(array=w454, index=w459, length=w457) -> (w453:dbl[])
                      n246 = Array Size(array=w453) -> (size(s)=w452:i32)
                      n247 = Divide(x=w452, y=2) -> (x/y=w462:dbl)
                      n248 = Round Toward -Infinity(1:w462) -> (0:w461:dbl)
                      n249 = Array Subset(array=w453, index=w461) -> (w474:dbl[])  [unwired: 1 in]
                      "subarray 2" <- w474
                      n250 = Array Subset(array=w453, index=0, length=w461) -> (w466:dbl[])
                      n251 = Add Array Elements(numeric array=w474) -> (sum=w479:dbl)
                      n252 = Add Array Elements(numeric array=w466) -> (sum=w470:dbl)
                      n253 = Array Size(array=w474) -> (size(s)=w464:i32)
                      n254 = Array Size(array=w466) -> (size(s)=w463:i32)
                      n255 = Divide(x=w479, y=w464) -> (x/y=w480:dbl)
                      n256 = Divide(x=w470, y=w463) -> (x/y=w469:dbl)
                      n257 = Divide(x=w480, y=65535.0) -> (x/y=w481:dbl)
                      n258 = Divide(x=w469, y=65535.0) -> (x/y=w468:dbl)
                      n259 = Multiply(x=w481, y=470.0) -> (x*y=w482:dbl)
                      n260 = Multiply(x=w468, y=470.0) -> (x*y=w467:dbl)
                      n261 = Add(x=w482, y=30.0) -> (x+y=w449:dbl)
                      n262 = Add(x=w467, y=30.0) -> (x+y=w450:dbl)
                    }
                  }
                  "sensor2-2 dis" <- w436
                  "x+y 2" <- w435
                }
                frame #1 {
                  n263 = Initialize Array(0.0 ("element"), w487) -> (w489:dbl[])
                  n264 = Replace Array Subset(array=w486, new element=w489) -> (w485:dbl[])  [unwired: 1 in]
                }
              }
            }
            frame True {
              n265 = flat-sequence {
                tunnel: w496 -> [w499]
                tunnel: [w499] -> w495
                tunnel: [w498] -> w494
                tunnel: [w497] -> w492
                tunnel: w495 -> [w530]
                tunnel: w494 -> [w529]
                tunnel: [w528] -> w493
                tunnel: [w527] -> w491
                tunnel: w492 -> [w527]
                frame #0 {
                  n266 = Search 1D Array(1D array=w499, element=0.0) -> (index of element=w503:i32)  [unwired: 1 in]
                  n267 = Array Size(array=w499) -> (size(s)=w498:i32)
                  n268 = Equal?(x=w503, y=-1) -> (x = y?=w505:bool)
                  n269 = Select(t=w498, s=w505, f=w503) -> (s? t:f=w504:i32)
                  n270 = Array Subset(array=w499, index=0, length=w504) -> (w502:dbl[])
                  n271 = Array Size(array=w502) -> (size(s)=w501:i32)
                  n272 = Greater Than 0?(x=w501) -> (x > 0?=w500:bool)
                  n273 = case shown="True" w500 {
                    tunnel: w502 -> [_ w526]
                    tunnel: w501 -> [_ w525]
                    tunnel: [200.0 w510] -> w497
                    frame False {
                    }
                    frame True {
                      n274 = Multiply(x=w525, y=0.25) -> (x*y=w516:dbl)
                      n275 = Multiply(x=w525, y=0.75) -> (x*y=w514:dbl)
                      n276 = Round Toward -Infinity(1:w516) -> (0:w515:dbl)
                      n277 = Round Toward -Infinity(1:w514) -> (0:w512:dbl)
                      n278 = Array Subset(array=w526, index=w515, length=w512) -> (w511:dbl[])
                      n279 = Add Array Elements(numeric array=w511) -> (sum=w521:dbl)
                      n280 = Divide(x=w521, y=w525) -> (x/y=w522:dbl)
                      n281 = Divide(x=w522, y=65535.0) -> (x/y=w523:dbl)
                      n282 = Multiply(x=w523, y=470.0) -> (x*y=w524:dbl)
                      n283 = Add(x=w524, y=30.0) -> (x+y=w510:dbl)
                    }
                  }
                  "sensor2 dis" <- w497
                }
                frame #1 {
                  n284 = Initialize Array(0.0 ("element"), w529) -> (w532:dbl[])
                  n285 = Replace Array Subset(array=w530, new element=w532) -> (w528:dbl[])  [unwired: 1 in]
                }
              }
              n286 = property on="sensor2-2 dis" class="DigNum (strict)"() -> ("Value"=w490:dbl)  [unwired: 2 in, 2 out]
            }
          }
        }
        frame #1 {
          n287 = Add(x=w659, y=w642) -> (x+y=w665:dbl)
          n288 = Add(x=w658, y=w641) -> (x+y=w666:dbl)
          n289 = Divide(x=w665, y=2.0) -> (x/y=w649:dbl)
          n290 = Divide(x=w666, y=2.0) -> (x/y=w648:dbl)
          n291 = Subtract(x=w649, y=w640) -> (x-y=w654:dbl)
          n292 = Subtract(x=w648, y=w639) -> (x-y=w652:dbl)
          n293 = Add(x=w654, y="bias") -> (x+y=w653:dbl)
          n294 = Add(x=w652, y="bias") -> (x+y=w650:dbl)
          n295 = case shown="0, Default" w661 {
            tunnel: w660 -> [w745 w759 w766 w774]
            tunnel: w661 -> [_ w758 w765 w773]
            tunnel: w653 -> [w744 w757 w764 w772]
            tunnel: [w736 w748 w763 w771] -> w662
            tunnel: w650 -> [w741 _ _ _]
            tunnel: w647 -> [w734 w747 w762 w770]
            tunnel: [w689 w747 w762 w770] -> w646
            tunnel: w645 -> [w733 _ _ _]
            tunnel: [w688 dbl[] [0.0, 0.0, 0.0, 0.0, 0.0] ("Col Curve 2") dbl[] [0.0, 0.0, 0.0, 0.0, 0.0] ("Col Curve 2") dbl[] [0.0, 0.0, 0.0, 0.0, 0.0] ("Col Curve 2")] -> w644
            tunnel: w643 -> [w687 _ _ _]
            frame 0, Default {
              n296 = Replace Array Subset(array=w745, new element #1=w744, index #1=5 ("index"), new element #2=w741, index #2=0 ("index")) -> (w736:dbl[])
              n297 = Array Subset(array=w736, index=1) -> (w739:dbl[])  [unwired: 1 in]
              n298 = Reshape Array(w739, 1 ("dimension size"), 5 ("dimension size")) -> (w735:dbl[][])
              n299 = call "curv avg.vi"("curv avg array in"=w734, "5 col curv"=w735, "sen plt num"=w733) -> ("curv avg array out"=w689:dbl[][][])  [unwired: 16 in]
              n300 = Array Size(array=w689) -> (size(s)=w700:i32[])
              n301 = Array Subset(array=w689, index (dim 0)=w687, length (dim 0)=1 ("length")) -> (w732:dbl[][][])  [unwired: 4 in]
              n302 = Index Array(array=w700, index #1=1 ("index"), index #2=2 ("index")) -> (element #1=w699:i32, element #2=w698:i32)
              n303 = Reshape Array(w732, w699, w698) -> (w731:dbl[][])
              n304 = Index Array(array=w731, index (col) #1=0 ("disabled index (col)"), index (col) #2=1 ("index (col)"), index (col) #3=2 ("index (col)"), index (col) #4=3 ("index (col)"), index (col) #5=4 ("index (col)")) -> (element #1=w727:dbl[], element #2=w718:dbl[], element #3=w717:dbl[], element #4=w716:dbl[], element #5=w715:dbl[])  [unwired: 5 in]
              n305 = Add Array Elements(numeric array=w727) -> (sum=w714:dbl)
              n306 = Equal To 0?(x=w727) -> (x = 0?=w730:bool[])
              n307 = Add Array Elements(numeric array=w718) -> (sum=w706:dbl)
              n308 = Equal To 0?(x=w718) -> (x = 0?=w725:bool[])
              n309 = Add Array Elements(numeric array=w717) -> (sum=w707:dbl)
              n310 = Equal To 0?(x=w717) -> (x = 0?=w724:bool[])
              n311 = Add Array Elements(numeric array=w716) -> (sum=w708:dbl)
              n312 = Equal To 0?(x=w716) -> (x = 0?=w721:bool[])
              n313 = Add Array Elements(numeric array=w715) -> (sum=w709:dbl)
              n314 = Equal To 0?(x=w715) -> (x = 0?=w720:bool[])
              n315 = Boolean To (0,1)(Boolean=w730) -> (0, 1=w729:i16[])
              n316 = Boolean To (0,1)(Boolean=w725) -> (0, 1=w710:i16[])
              n317 = Boolean To (0,1)(Boolean=w724) -> (0, 1=w711:i16[])
              n318 = Boolean To (0,1)(Boolean=w721) -> (0, 1=w712:i16[])
              n319 = Boolean To (0,1)(Boolean=w720) -> (0, 1=w713:i16[])
              n320 = Add Array Elements(numeric array=w729) -> (sum=w728:i16)
              n321 = Add Array Elements(numeric array=w710) -> (sum=w726:i16)
              n322 = Add Array Elements(numeric array=w711) -> (sum=w723:i16)
              n323 = Add Array Elements(numeric array=w712) -> (sum=w722:i16)
              n324 = Add Array Elements(numeric array=w713) -> (sum=w719:i16)
              n325 = Subtract(x=w699, y=w728) -> (x-y=w685:i32)
              n326 = Subtract(x=w699, y=w726) -> (x-y=w680:i32)
              n327 = Subtract(x=w699, y=w723) -> (x-y=w676:i32)
              n328 = Subtract(x=w699, y=w722) -> (x-y=w672:i32)
              n329 = Subtract(x=w699, y=w719) -> (x-y=w668:i32)
              n330 = Equal To 0?(x=w685) -> (x = 0?=w686:bool)
              n331 = Equal To 0?(x=w680) -> (x = 0?=w681:bool)
              n332 = Equal To 0?(x=w676) -> (x = 0?=w678:bool)
              n333 = Equal To 0?(x=w672) -> (x = 0?=w673:bool)
              n334 = Equal To 0?(x=w668) -> (x = 0?=w670:bool)
              n335 = Select(t=1, s=w686, f=w685) -> (s? t:f=w683:i32)
              n336 = Select(t=1, s=w681, f=w680) -> (s? t:f=w679:i32)
              n337 = Select(t=1, s=w678, f=w676) -> (s? t:f=w675:i32)
              n338 = Select(t=1, s=w673, f=w672) -> (s? t:f=w671:i32)
              n339 = Select(t=1, s=w670, f=w668) -> (s? t:f=w667:i32)
              n340 = Divide(x=w714, y=w683) -> (x/y=w705:dbl)
              n341 = Divide(x=w706, y=w679) -> (x/y=w704:dbl)
              n342 = Divide(x=w707, y=w675) -> (x/y=w703:dbl)
              n343 = Divide(x=w708, y=w671) -> (x/y=w702:dbl)
              n344 = Divide(x=w709, y=w667) -> (x/y=w701:dbl)
              n345 = Build Array(w705, w704, w703, w702, w701) -> (w688:dbl[])
            }
            frame 1 {
              w749 = 0.0 ("new element/subarray")
              n346 = Increment(x=w758) -> (x+1=w760:dbl)
              n347 = Replace Array Subset(array=w759, new element=w757, index=w760) -> (w755:dbl[])
              n348 = Index Array(array=w755, index=0) -> (element=w753:dbl)
              n349 = Replace Array Subset(array=w755, new element #1=w753, index #1=1 ("index"), new element #2=w749, index #2=3 ("index"), new element #3=w749, index #3=4 ("index"), new element #4=w749, index #4=5 ("index")) -> (w748:dbl[])
            }
            frame 2 {
              n350 = Increment(x=w765) -> (x+1=w767:dbl)
              n351 = Replace Array Subset(array=w766, new element=w764, index=w767) -> (w763:dbl[])
            }
            frame 3 {
              n352 = Increment(x=w773) -> (x+1=w775:dbl)
              n353 = Replace Array Subset(array=w774, new element=w772, index=w775) -> (w771:dbl[])
              "Boolean" <- FALSE
            }
          }
          "curv array in 2" <- w662
        }
      }
    }
  }
  "curv array out" <- w83
  "sensor1 array out" <- w65
  "sensor2 array out" <- w64
  "sensor3 array out" <- w63
  "cyrv avg array out" <- w45
  "Col Curve" <- w41
  n354 = Array Max & Min(array=w41) -> (max value=w86:dbl)  [unwired: 3 out]
  "Pallet CURV (mm)" <- w86
  n355 = Greater Or Equal?(x=w86, y=w43) -> (x >= y?=→"curv sit":bool)
